vi "Thermo Analyzers Example 1.vi"() -> ()   [LabVIEW 2010]
uses:
  <vilib>/Analysis/Matrix/Datatypes/RealMatrix.ctl
  <vilib>/Analysis/Matrix/NI_Matrix.lvlib
panel:
  in  "Frequency (Hz)":dbl=0.1
  out "Data Out":T1(array[cluster])
  out "error out":errorcluster
  out "Thermo Analyzer Data":dbl[][](graph)
  in  "Stop Button":bool
  in  "Instrument":T2(ring)
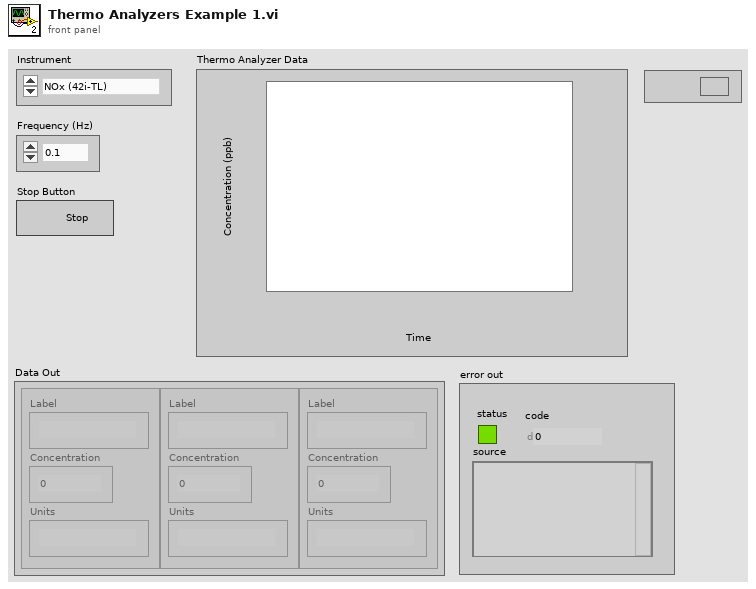
[diagram p1: front panel]
types:
  T1 = cluster{"Label":string, "Concentration":sgl, "Units":string}[]
  T2 = enum16{"NOx (42i-TL)", "SO2 (43i-TLE)", "O3 (49i)"}
  T3 = typedef "NI_Matrix.lvlib/RealMatrix.ctl" = dbl[][]
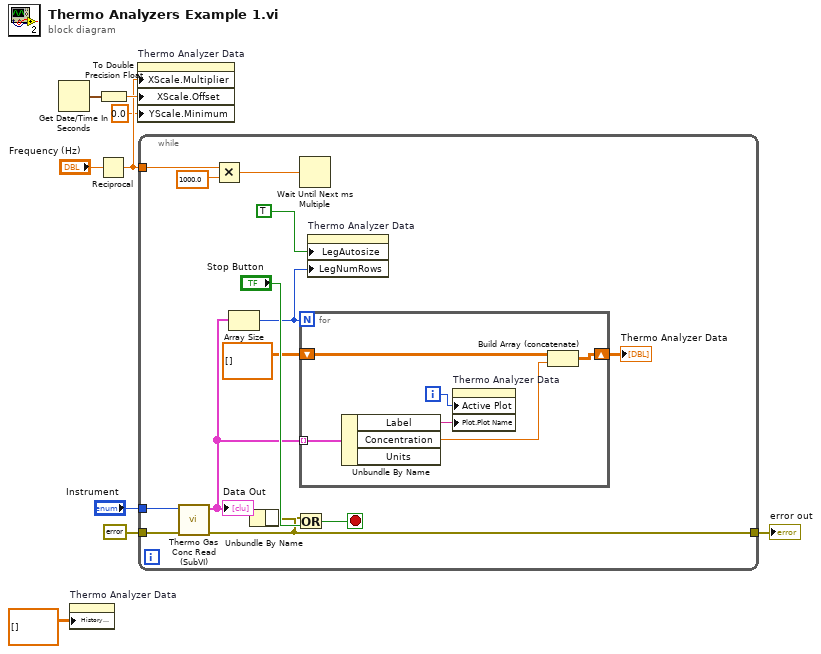
[diagram p0: block diagram]
diagram:
  n1 = Get Date/Time In Seconds() -> (seconds since 1Jan1904=w5:timestamp)
  n2 = property on="Thermo Analyzer Data" class="WFChart (strict)"("History Data"=dbl[][] []) -> ()  [unwired: 2 in, 2 out]
  n3 = Reciprocal(x="Frequency (Hz)") -> (1/x=w3:dbl)
  n4 = To Double Precision Float(number=w5) -> (double precision float=w4:dbl)
  n5 = property on="Thermo Analyzer Data" class="WFChart (strict)"("XScale.Multiplier"=w3, "XScale.Offset"=w4, "YScale.Minimum"=0.0 ("Y Scale.Range:Minimum")) -> ()  [unwired: 2 in, 2 out]
  n6 = while {
    tunnel: "Instrument" -> [w11]
    tunnel: errorcluster {"status"=FALSE, "code"=0, "source"=""} ("Error In") -> [w23]
    tunnel: [w20] -> w7
    tunnel: w3 -> [w17]
    stop <- w22 stop-if-true
    n7 = call "Thermo Gas Conc Read (SubVI).vi"("Error In"=w23, "Instrument"=w11) -> ("error out"=w20:errorcluster, "Data Out"=w14:T1)  [unwired: 8 in]
    "Data Out" <- w14
    n8 = Multiply(x=w17, y=1000.0) -> (x*y=w16:dbl)
    n9 = Array Size(array=w14) -> (size(s)=w12:i32)
    n10 = Or(y="Stop Button") -> (x=w10:errorcluster, x .or. y?=w22:bool)
    n11 = Unbundle By Name(w20, w10) -> ()
    n12 = Wait Until Next ms Multiple(millisecond multiple=w16) -> ()  [unwired: 1 out]
    n13 = for {
      N: w12 -> [_]
      tunnel: w14 -> [w29] mode=indexing
      shift-right: [w28] -> w19
      shift-left: T3 [] ("Real Matrix") -> [w26]
      i -> [w25]
      n14 = Unbundle By Name(w29) -> ("Label"=w24:string, "Concentration"=w27:sgl)  [unwired: 1 out]
      n15 = property on="Thermo Analyzer Data" class="WFChart (strict)"("Active Plot"=w25, "Plot.Plot Name"=w24) -> ()  [unwired: 2 in, 2 out]
      n16 = Build Array (concatenate)(w26, w27) -> (w28:T3)
    }
    "Thermo Analyzer Data" <- w19
    n17 = property on="Thermo Analyzer Data" class="WFChart (strict)"("LegAutosize"=TRUE ("Legend:Autosize"), "LegNumRows"=w12) -> ()  [unwired: 2 in, 2 out]
  }
  "error out" <- w7
